vi "Sum channels.vi"(1 "Count in":i32[][](array[numeric]), 2 "scale":dbl=1.0) -> (0 "Count out":i32[][](array[numeric]))   [LabVIEW 2014]
panel:
  # "sums row into last row element for 8xn data array"
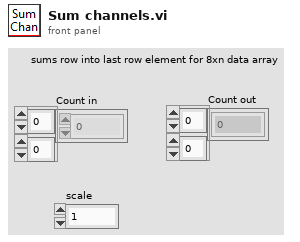
[diagram p1: front panel]
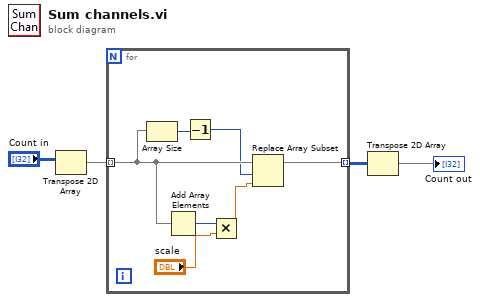
[diagram p0: block diagram]
diagram:
  n1 = Transpose 2D Array(2D array="Count in") -> (transposed array=w3:i32[][])
  n2 = for {
    tunnel: w3 -> [w10] mode=indexing
    tunnel: [w11] -> w2 mode=indexing
    n3 = Array Size(array=w10) -> (size(s)=w8:i32)
    n4 = Add Array Elements(numeric array=w10) -> (sum=w7:i32)
    n5 = Decrement(x=w8) -> (x-1=w9:i32)
    n6 = Multiply(x=w7, y="scale") -> (x*y=w6:dbl)
    n7 = Replace Array Subset(array=w10, new element=w6, index=w9) -> (w11:i32[])
  }
  n8 = Transpose 2D Array(2D array=w2) -> (transposed array=→"Count out":i32[][])
